vi "DB -Path.vi"(11 "path":path) -> (1 "String 3":string, 2 "String 2":string, 3 "String":string)   [LabVIEW 2024]
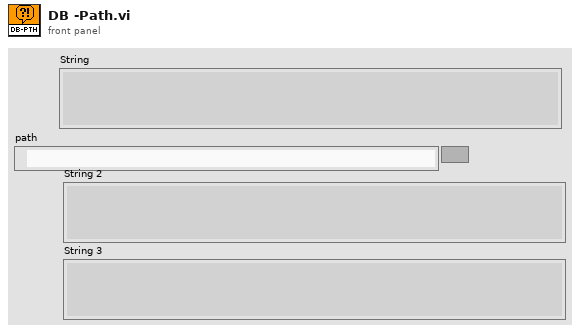
[diagram p1: front panel]
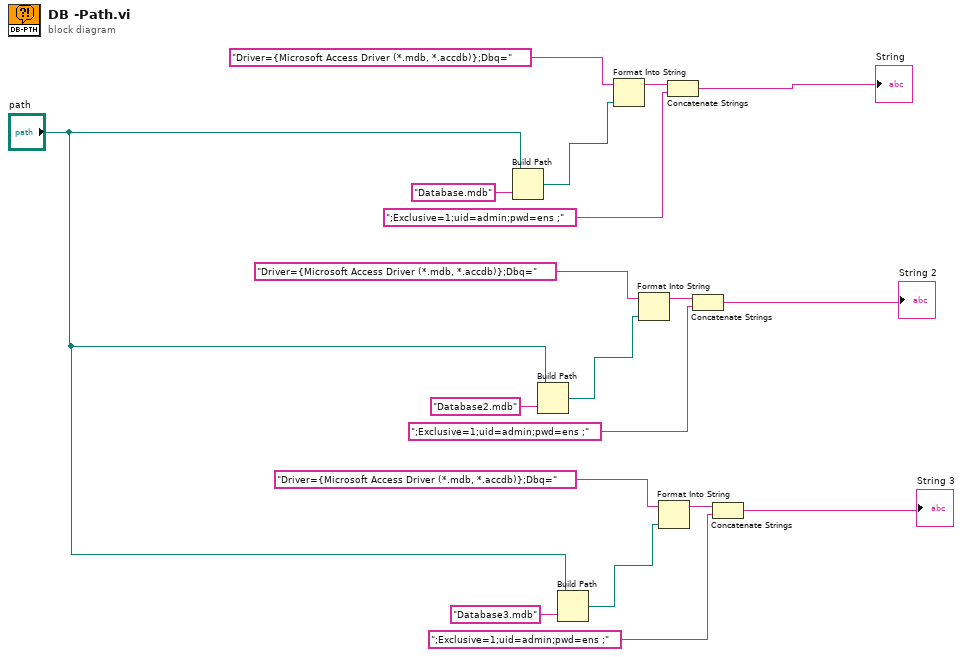
[diagram p0: block diagram]
diagram:
  n1 = Build Path(base path="path", name or relative path="Database.mdb") -> (appended path=w14:path)
  n2 = Build Path(base path="path", name or relative path="Database2.mdb") -> (appended path=w13:path)
  n3 = Build Path(base path="path", name or relative path="Database3.mdb") -> (appended path=w4:path)
  n4 = Format Into String(initial string="Driver={Microsoft Access Driver (*.mdb, *.accdb)};Dbq=" ("name or relative path"), w14) -> (resulting string=w17:string)  [unwired: 2 in, 1 out]
  n5 = Format Into String(initial string="Driver={Microsoft Access Driver (*.mdb, *.accdb)};Dbq=" ("name or relative path"), w13) -> (resulting string=w10:string)  [unwired: 2 in, 1 out]
  n6 = Format Into String(initial string="Driver={Microsoft Access Driver (*.mdb, *.accdb)};Dbq=" ("name or relative path"), w4) -> (resulting string=w7:string)  [unwired: 2 in, 1 out]
  n7 = Concatenate Strings(w17, ";Exclusive=1;uid=admin;pwd=ens ;") -> (→"String":string)
  n8 = Concatenate Strings(w10, ";Exclusive=1;uid=admin;pwd=ens ;") -> (→"String 2":string)
  n9 = Concatenate Strings(w7, ";Exclusive=1;uid=admin;pwd=ens ;") -> (→"String 3":string)
